vi "Write Array of Motor Category Strings.vi"(8 "error in (no error)":errorcluster, 10 "Array of Category Strings":string[](array[string]), 11 "MotionSystem Configuration in":refnum<class "MotionSystem Configuration.lvclass">) -> (0 "error out":errorcluster, 3 "MotionSystem Configuration out":refnum<class "MotionSystem Configuration.lvclass">)   [LabVIEW 2016, in "MotionSystem.lvlib" / "MotionSystem Configuration.lvclass"]
uses:
  <userlib>/Common Components/Hardware/Abstract System/MotionSystem/MotionSystem Config/MotionSystem Configuration.lvclass
  <userlib>/Common Components/Hardware/Abstract System/MotionSystem/MotionSystem Config/MotionSystem Configuration.lvclass/MotionSystem Configuration.ctl
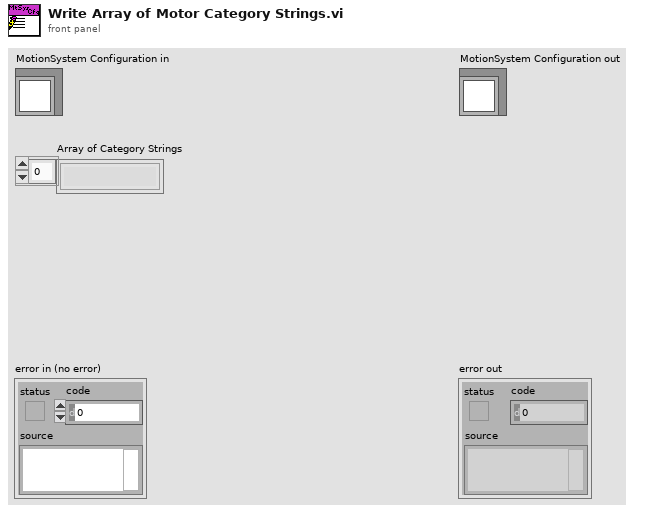
[diagram p1: front panel]
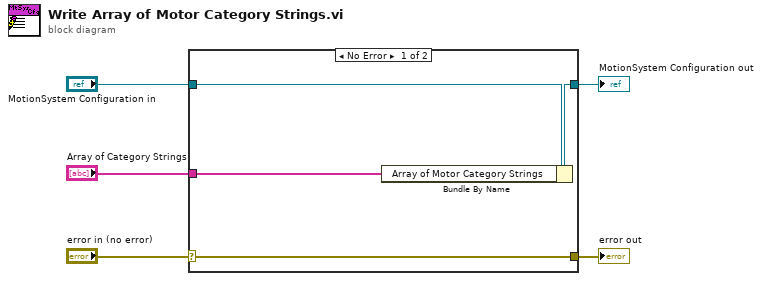
[diagram p0: block diagram]
diagram:
  n1 = case shown="No Error" "error in (no error)" {
    selector: "error in (no error)" -> [w9 w10]
    tunnel: [w9 w10] -> w4
    tunnel: [w7 w11] -> w2
    tunnel: "MotionSystem Configuration in" -> [w8 w11]
    tunnel: "Array of Category Strings" -> [w6 _]
    frame No Error {
      n2 = Bundle By Name(cluster=w8, "Array of Motor Category Strings"=w6) -> (w7:refnum<class "MotionSystem Configuration.lvclass">)
    }
    frame Error {
    }
  }
  "error out" <- w4
  "MotionSystem Configuration out" <- w2
